vi "Measurement Parser.vi"(7 "Waveform Graph":dynamicdata(graph), 8 "error in (no error)":errorcluster, 9 "Generic Card in":refnum<class "Generic Card.lvclass">, 10 "Data Array":dbl[](array[numeric]), 11 "Tektronix PA1000 in":refnum<class "Tektronix PA1000.lvclass">) -> (0 "error out":errorcluster, 3 "Tektronix PA1000 out":refnum<class "Tektronix PA1000.lvclass">)   [LabVIEW 2014, in "Generic Power Analyzer.lvlib" / "Tektronix PA1000.lvlib" / "Tektronix PA1000.lvclass"]
uses:
  Tektronix PA1000.lvclass
  Generic Instrument/Generic Card/Generic Card.lvclass
  Generic Power Analyzer/Generic Power Analyzer.lvclass
  <instrlib>/Tektronix PA1000/Tektronix PA1000.lvlib
  Data Logger/Data Logger.lvclass
panel:
  out "Numeric":dbl
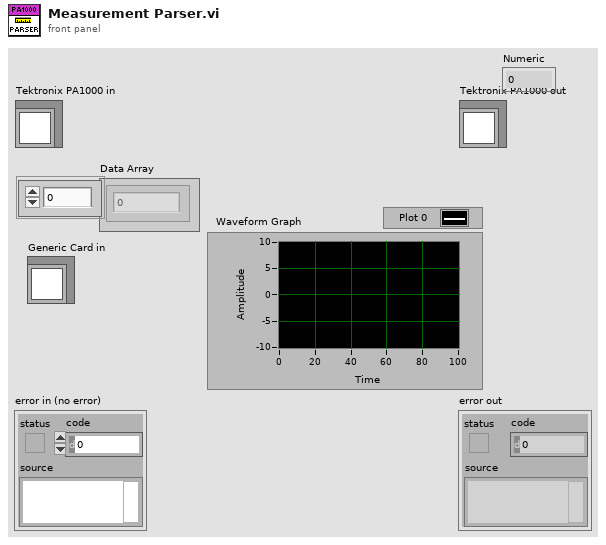
[diagram p1: front panel]
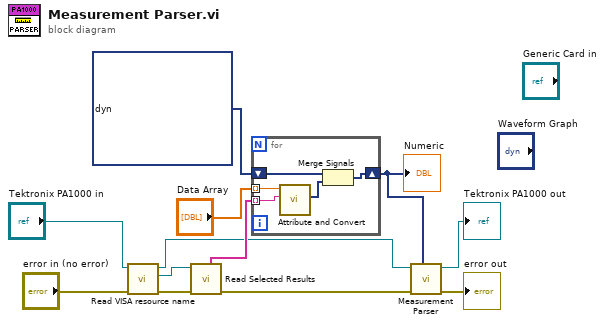
[diagram p0: block diagram]
diagram:
  n1 = call-dynamic "Read VISA resource name.vi"("error in (no error)"="error in (no error)", "Generic Instrument in"="Tektronix PA1000 in") -> ("error out"=w9:errorcluster, "VISA resource name"=w10:refnum<visa-resource-name>, "Generic Instrument out"=w8:refnum<class "Tektronix PA1000.lvclass">)  [unwired: 7 in]
  n2 = call <instrlib>:"Read Selected Results.vi"("error in (no error)"=w9, "VISA resource name"=w10) -> ("error out"=w4:errorcluster, "Measurement List"=w12:string[])  [unwired: 5 in, 3 out]
  n3 = for {
    tunnel: "Data Array" -> [w14] mode=indexing
    tunnel: w12 -> [w17] mode=indexing
    shift-right: [w13] -> w1
    shift-left: dynamicdata [] ("Waveform Graph 2") -> [w16]
    n4 = call "Attribute and Convert.vi"("Signal Name"=w17, "Number in"=w14) -> ("Dynamic Signal Out"=w15:dynamicdata)  [unwired: 9 in]
    n5 = Merge Signals(w16, w15) -> (w13:dynamicdata)
  }
  "Numeric" <- w1
  n6 = call-parent "Measurement Parser.vi"("Waveform Graph"=w1, "error in (no error)"=w4, "Generic Power Analyzer in"=w8) -> ("error out"=→"error out":errorcluster, "Generic Power Analyzer out"=→"Tektronix PA1000 out":refnum<class "Tektronix PA1000.lvclass">)  [unwired: 7 in]
